vi "FTW-Test-Array-Shuffle.vi"() -> (0 "Test Result":errorcluster)   [LabVIEW 2014]
uses:
  src/core/error/FTW-ERR-ThrowError.vi
  src/core/error/FTW-ERR-CallChain.vi
  src/core/string/FTW-STR-ReplaceWhitespace.vi
  src/core/array/shuffle/FTW-Array-Shuffle.xnode
panel:
  out "Slope of Regression Line":dbl
  out "Differentials":dbl[](graph)
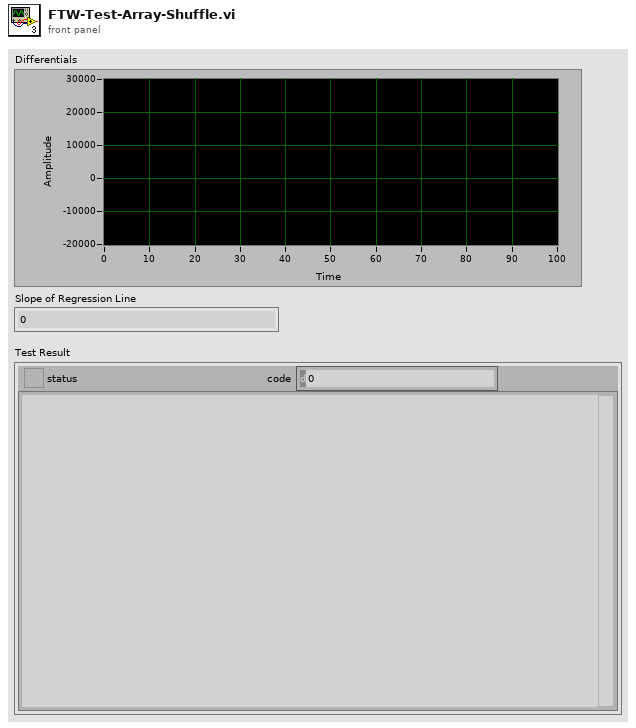
[diagram p1: front panel]
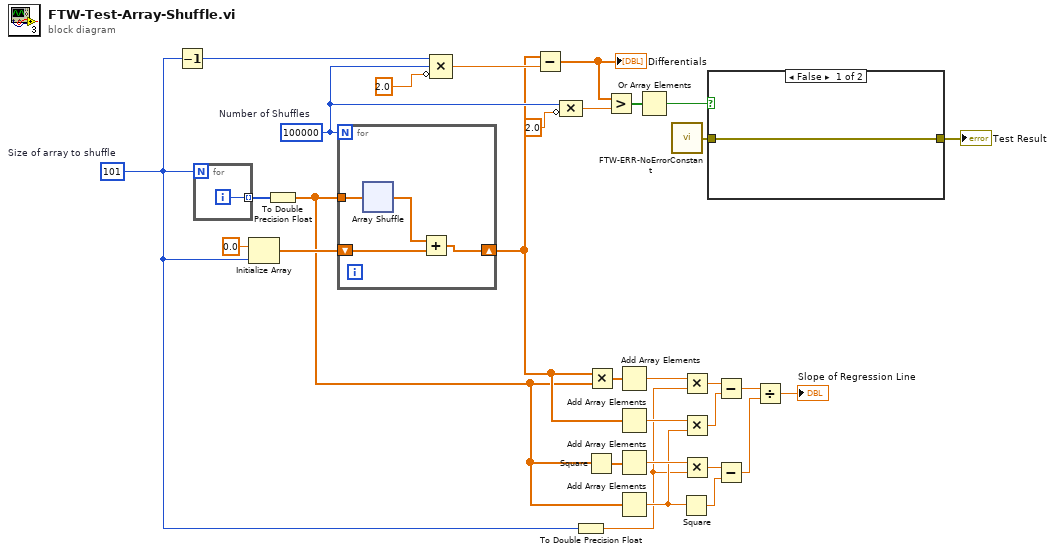
[diagram p0: block diagram]
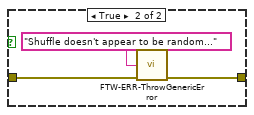
[diagram p2: hidden frame]
diagram:
  w23 = 100000  # Number of Shuffles
  w8 = 101  # Size of array to shuffle
  n1 = Decrement(x=w8) -> (x-1=w28:i32)
  n2 = for {
    N: w8 -> [_]
    tunnel: [w32] -> w29 mode=indexing
    i -> [w32]
  }
  n3 = Initialize Array(0.0 ("element"), w8) -> (w30:dbl[])
  n4 = To Double Precision Float(number=w29) -> (double precision float=w11:dbl[])
  n5 = for {
    N: w23 -> [_]
    shift-right: [w34] -> w15
    shift-left: w30 -> [w35]
    tunnel: w11 -> [w33]
    n6 = xnode "Array Shuffle"("Array"=w33) -> ("Shuffled Array"=w36:dbl[])
    n7 = Add(x=w36, y=w35) -> (x+y=w34:dbl[])
  }
  n8 = Compound Arithmetic op=MULTIPLY(w28, w23, invert 2.0) -> (w26:dbl)
  n9 = Subtract(x=w15, y=w26) -> (x-y=w25:dbl[])
  "Differentials" <- w25
  n10 = Compound Arithmetic op=MULTIPLY(w23, invert 2.0) -> (w22:dbl)
  n11 = To Double Precision Float(number=w8) -> (double precision float=w1:dbl)
  n12 = Square(x=w11) -> (x^2=w10:dbl[])
  n13 = Multiply(x=w15, y=w11) -> (x*y=w17:dbl[])
  n14 = Greater?(x=w25, y=w22) -> (0:w24:bool[])
  n15 = Add Array Elements(numeric array=w17) -> (sum=w16:dbl)
  n16 = Add Array Elements(numeric array=w15) -> (sum=w14:dbl)
  n17 = Add Array Elements(numeric array=w10) -> (sum=w9:dbl)
  n18 = Add Array Elements(numeric array=w11) -> (sum=w6:dbl)
  n19 = Or Array Elements(Boolean array=w24) -> (logical OR=w19:bool)
  n20 = call "FTW-ERR-NoErrorConstant.vi"() -> ("no error"=w18:errorcluster)
  n21 = Square(x=w6) -> (x^2=w5:dbl)
  n22 = Multiply(x=w16, y=w1) -> (x*y=w13:dbl)
  n23 = Multiply(x=w14, y=w6) -> (x*y=w12:dbl)
  n24 = Multiply(x=w9, y=w1) -> (x*y=w4:dbl)
  n25 = case shown="False" w19 {
    tunnel: [w54 w57] -> w20
    tunnel: w18 -> [w54 w55]
    frame False {
    }
    frame True {
      n26 = call "FTW-ERR-ThrowGenericError.vi"("Error Message"="Shuffle doesn't appear to be random...", "error in"=w55) -> ("error out"=w57:errorcluster)  [unwired: 13 in]
    }
  }
  "Test Result" <- w20
  n27 = Subtract(x=w13, y=w12) -> (x-y=w7:dbl)
  n28 = Subtract(x=w4, y=w5) -> (x-y=w3:dbl)
  n29 = Divide(x=w7, y=w3) -> (x/y=→"Slope of Regression Line":dbl)
